vi "SplitClassic.vi"(8 "error in (no error)":errorcluster caption="entrée d'erreur (pas d'erreur)", 9 "Y":string[][](array[string]), 10 "X":string[][](array[string]), 11 "TestTrain":T2={"test_size"=-1.0, "train_size"=-1.0, "random_state"=-1, "shuffle"=TRUE, "stratify"=[]} {"random_state" min=-1; "train_size" min=-1.0; "test_size" min=-1.0}) -> (0 "error out":errorcluster caption="sortie d'erreur", 1 "Y_Test":T1, 2 "X_Train":T1, 3 "X_Test":T1, 4 "Y_Train":T1)   [LabVIEW 2020]
doc: "Split arrays or matrices into random train and test subsets\n\nQuick utility that wraps input validation and next(ShuffleSplit().split(X, y)) and application to input data into a single call for splitting (and optionally subsampling) data in a oneliner.\n\n\nParameters : \n\n- test_size : float or int, default=None=-1\nIf float, should be between 0.0 and 1.0 and represent the proportion of the dataset to include in the test split. If int, represents the absolute number of test samples. If None, the value is set to the complement of the train size. If train_size is also None, it will be set to 0.25.\n\n- train_size : float or int, default=None=-1\nIf float, should be between 0.0 and 1.0 and represent the proportion of the dataset to include in the train split. If int, represents the absolute number of train samples. If None, the value is automatically set to the complement of the test size.\n\n- random_stateint or RandomState instance, default=None=-1\nControls the shuffling applied to the data before applying the split. Pass an int for reproducible output across multiple function calls. See Glossary.\n\n- shuffle : bool, default=True\nWhether or not to shuffle the data before splitting. If shuffle=False then stratify must be None.\n\n- stratify : array-like, default=None\nIf not None, data is split in a stratified fashion, using this as the class labels.\n\nReturns : \n\n- splitting : list, length=2 * len(arrays)\nList containing X_Test split of inputs."
uses:
  TrainTest.lvclass
panel:
  out "TrainTest.lvclass":refnum<class "TrainTest.lvclass">
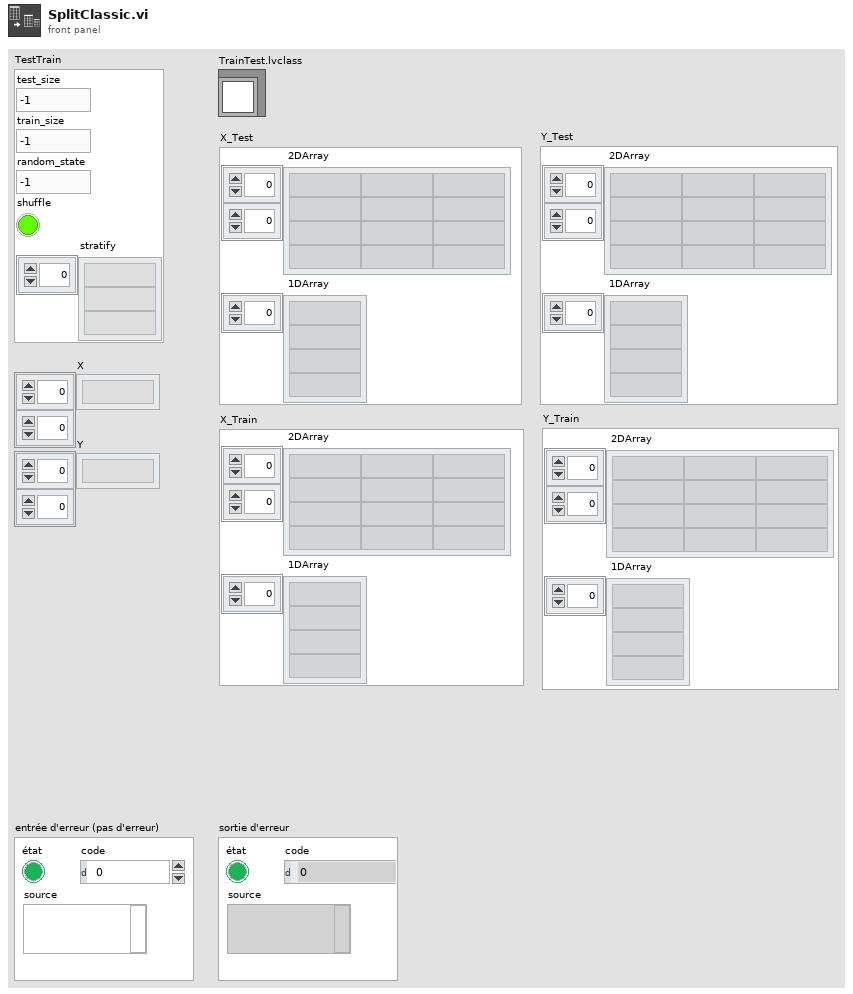
[diagram p1: front panel]
types:
  T1 = cluster{" 4DArray":cluster{"1":string[][], "2":string[][]}[], " 3DArray":cluster{"Tableau":string[][]}[], "Sparse Matrix 2DArray":string[][], " 2DArray":string[][], " 1DArray":string[]}
  T2 = cluster{"test_size":dbl, "train_size":dbl, "random_state":i32, "shuffle":bool, "stratify":string[]}
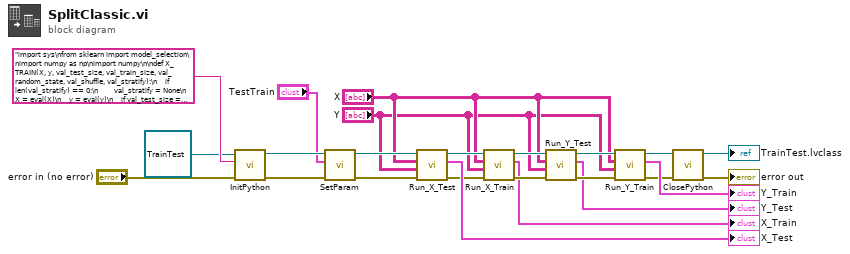
[diagram p0: block diagram]
diagram:
  n1 = call-dynamic "InitPython.vi"("error in (no error)"="error in (no error)", "Python Instruction"="import sys\nfrom sklearn import model_selection\nimport numpy as np\nimport numpy\n\ndef X_TRAIN(X, y, val_test_size, val_train_size, val_random_state, val_shuffle, val_stratify):\n    if len(val_stratify) == 0:\n        val_stratify = None\n    X = eval(X)\n    y = eval(y)\n    if val_test_size == -1:\n        val_test_size = None\n    if val_train_size == -1:\n        val_train_size = None\n    if val_random_state == -1:\n        val_random_state = None\n    try:\n        X_train, X_test, y_train, y_test= model_selection.train_test_split(X, y, test_size=val_test_size, train_size=val_train_size, random_state=val_random_state, shuffle=val_shuffle, stratify=val_stratify)\n        return str(X_train)\n    except:\n        erreur = sys.exc_info()\n        typerr = u\"%s\" % (erreur[0])\n        typerr = typerr[typerr.find(\"'\")+1:typerr.rfind(\"'\")]\n        msgerr = u\"%s\" % (erreur[1])\n        message = str('/!\\\\ {0} : {1}'. format(typerr,msgerr))\n        return message \n\ndef X_TEST(X, y, val_test_size, val_train_size, val_random_state, val_shuffle, val_stratify):\n    if len(val_stratify) == 0:\n        val_stratify = None\n    X = eval(X)\n    y = eval(y)\n    if val_test_size == -1:\n        val_test_size = None\n    if val_train_size == -1:\n        val_train_size = None\n    if val_random_state == -1:\n        val_random_state = None\n    try:\n        X_train, X_test, y_train, y_test= model_selection.train_test_split(X, y, test_size=val_test_size, train_size=val_train_size, random_state=val_random_state, shuffle=val_shuffle, stratify=val_stratify)\n        return str(X_test)\n    except:\n        erreur = sys.exc_info()\n        typerr = u\"%s\" % (erreur[0])\n        typerr = typerr[typerr.find(\"'\")+1:typerr.rfind(\"'\")]\n        msgerr = u\"%s\" % (erreur[1])\n        message = str('/!\\\\ {0} : {1}'. format(typerr,msgerr))\n        return message\n    \ndef Y_TRAIN(X, y, val_test_size, val_train_size, val_random_state, val_shuffle, val_stratify):\n    if len(val_stratify) == 0:\n        val_stratify = None\n    X = eval(X)\n    y = eval(y)\n    if val_test_size == -1:\n        val_test_size = None\n    if val_train_size == -1:\n        val_train_size = None\n    if val_random_state == -1:\n        val_random_state = None\n    try:\n        X_train, X_test, y_train, y_test= model_selection.train_test_split(X, y, test_size=val_test_size, train_size=val_train_size, random_state=val_random_state, shuffle=val_shuffle, stratify=val_stratify)\n        return str(y_train)\n    except:\n        erreur = sys.exc_info()\n        typerr = u\"%s\" % (erreur[0])\n        typerr = typerr[typerr.find(\"'\")+1:typerr.rfind(\"'\")]\n        msgerr = u\"%s\" % (erreur[1])\n        message = str('/!\\\\ {0} : {1}'. format(typerr,msgerr))\n        return message\n    \ndef Y_TEST(X, y, val_test_size, val_train_size, val_random_state, val_shuffle, val_stratify):\n    if len(val_stratify) == 0:\n        val_stratify = None\n    X = eval(X)\n    y = eval(y)\n    if val_test_size == -1:\n        val_test_size = None\n    if val_train_size == -1:\n        val_train_size = None\n    if val_random_state == -1:\n        val_random_state = None\n    try:\n        X_train, X_test, y_train, y_test= model_selection.train_test_split(X, y, test_size=val_test_size, train_size=val_train_size, random_state=val_random_state, shuffle=val_shuffle, stratify=val_stratify)\n        return str(y_test)\n    except:\n        erreur = sys.exc_info()\n        typerr = u\"%s\" % (erreur[0])\n        typerr = typerr[typerr.find(\"'\")+1:typerr.rfind(\"'\")]\n        msgerr = u\"%s\" % (erreur[1])\n        message = str('/!\\\\ {0} : {1}'. format(typerr,msgerr))\n        return message", "Scikit-learn en entrée"=refnum<class "TrainTest.lvclass"> refnum ("TrainTest.lvclass")) -> ("error out"=w22:errorcluster, "Scikit-learn en sortie"=w21:refnum<class "TrainTest.lvclass">)  [unwired: 7 in]
  n2 = call-dynamic "SetParam.vi"("error in (no error)"=w22, "TestTrain"="TestTrain", "TrainTest.lvclass"=w21) -> ("error out"=w18:errorcluster, "TrainTest.lvclass"=w17:refnum<class "TrainTest.lvclass">)  [unwired: 7 in]
  n3 = call-dynamic "Run_X_Test.vi"("error in (no error)"=w18, "Y"="Y", "X"="X", "TrainTest.lvclass"=w17) -> ("error out"=w10:errorcluster, "Data"=→"X_Test":T1, "TrainTest.lvclass"=w15:refnum<class "TrainTest.lvclass">)  [unwired: 5 in]
  n4 = call-dynamic "Run_X_Train.vi"("error in (no error)"=w10, "Y"="Y", "X"="X", "TrainTest.lvclass"=w15) -> ("error out"=w11:errorcluster, "Data"=→"X_Train":T1, "TrainTest.lvclass"=w14:refnum<class "TrainTest.lvclass">)  [unwired: 5 in]
  n5 = call-dynamic "Run_Y_Test.vi"("error in (no error)"=w11, "Y"="Y", "X"="X", "TrainTest.lvclass 2"=w14) -> ("error out"=w12:errorcluster, "Data"=→"Y_Test":T1, "TrainTest.lvclass"=w13:refnum<class "TrainTest.lvclass">)  [unwired: 5 in]
  n6 = call-dynamic "Run_Y_Train.vi"("error in (no error)"=w12, "Y"="Y", "X"="X", "TrainTest.lvclass"=w13) -> ("error out"=w2:errorcluster, "Data"=→"Y_Train":T1, "TrainTest.lvclass"=w4:refnum<class "TrainTest.lvclass">)  [unwired: 5 in]
  n7 = call-dynamic "ClosePython.vi"("error in (no error)"=w2, "Scikit-learn en entrée"=w4) -> ("error out"=→"error out":errorcluster, "Scikit-learn en sortie"=→"TrainTest.lvclass":refnum<class "TrainTest.lvclass">)  [unwired: 8 in]
